vi "Clear Timing Override.vi"(8 "error in (no error)":errorcluster, 11 "CIFTemplateNode in":refnum<class "CIFTemplateNode.lvclass">) -> (0 "error out":errorcluster, 3 "CIFTemplateNode out":refnum<class "CIFTemplateNode.lvclass">)   [LabVIEW 2021, in "CIFTemplateNode.lvclass"]
uses:
  CIFTemplateNode.lvclass
  CIFTemplateNode.lvclass/CIFTemplateNode.ctl
  CIFTemplateCommon/Typedef/Timing Overrides.ctl
  CIFTemplateCommon/CIFTemplateCommon.lvlib
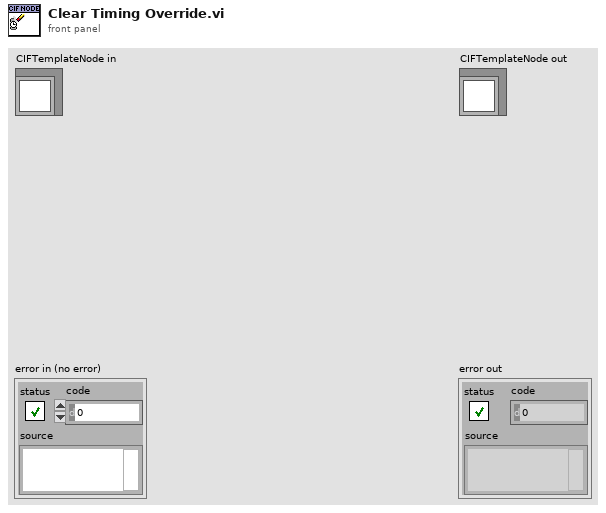
[diagram p1: front panel]
types:
  T1 = typedef "CIFTemplateCommon.lvlib/Timing Overrides.ctl" = cluster{"Override Timing":bool, "Period (s)":dbl}
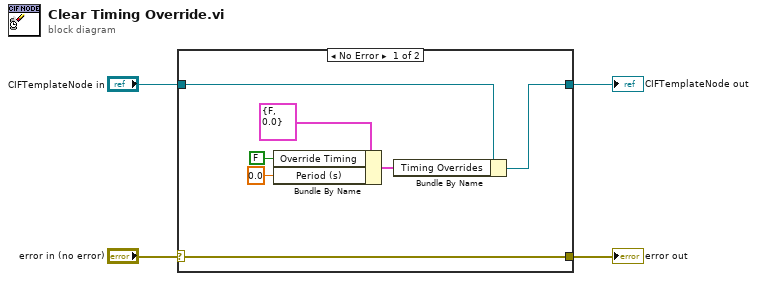
[diagram p0: block diagram]
diagram:
  n1 = case shown="No Error" "error in (no error)" {
    selector: "error in (no error)" -> [w11 w12]
    tunnel: [w11 w12] -> w3
    tunnel: [w9 w13] -> w1
    tunnel: "CIFTemplateNode in" -> [w10 w13]
    frame No Error {
      n2 = Bundle By Name(cluster=T1 {"Override Timing"=FALSE, "Period (s)"=0.0} ("Plugin Overrides.Timing Overrides"), "Override Timing"=FALSE, "Period (s)"=0.0) -> (w6:T1)
      n3 = Bundle By Name(cluster=w10, "Timing Overrides"=w6) -> (w9:refnum<class "CIFTemplateNode.lvclass">)
    }
    frame Error {
    }
  }
  "error out" <- w3
  "CIFTemplateNode out" <- w1
